vi "Format InstancePrivateIpAddressSetItemType_LVXML.vi"(8 "error in (no error)":errorcluster, 10 "valueXmlData 3":T2, 11 "AWS_EC2 in":refnum<class "AWS_EC2.lvclass">) -> (0 "error out":errorcluster, 2 "Array":T3[](array[typedef]), 3 "AWS_EC2 out":refnum<class "AWS_EC2.lvclass">)   [LabVIEW 2014, in "AWS_EC2.lvlib" / "AWS_EC2.lvclass"]
uses:
  AWS_EC2.lvclass
  EC2 Datatypes/InstancePrivateIpAddressesSetItemType.ctl
  EC2 Datatypes/InstanceNetworkInterfaceAssociationType.ctl
  lv-xml-parser/r0/trunk/VI Source/EventType.ctl
  lv-xml-parser/r0/trunk/VI Source/LV XML Parser.lvlib
  AWS_EC2.lvlib
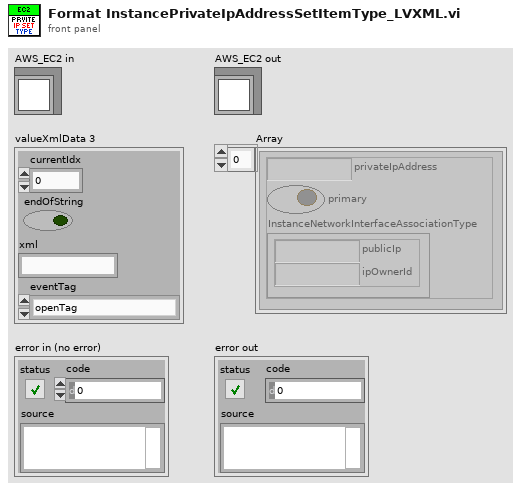
[diagram p1: front panel]
types:
  T1 = typedef "LV XML Parser.lvlib/EventType.ctl" = enum16{"openTag", "endOpenTag", "closeTag", "comment", "endComment", "endOfFile", "attribute", "startXml"}
  T2 = cluster{"currentIdx":i32, "endOfString":bool, "xml":string, "eventTag":T1}
  T3 = typedef "AWS_EC2.lvlib/InstancePrivateIpAddressesSetItemType.ctl" = cluster{"privateIpAddress":string, "primary":bool, "InstanceNetworkInterfaceAssociationType":T4}
  T4 = typedef "AWS_EC2.lvlib/InstanceNetworkInterfaceAssociationType.ctl" = cluster{"publicIp":string, "ipOwnerId":string}
  T5 = cluster{"namespaceUri":string, "localName":string}
  T6 = cluster{"Attributes":cluster{"localName":string, "namespaceUri":string, "value":string}[], "localName":string, "namespaceUri":string, "valueXmlData":cluster{"currentIdx":i32, "endOfString":bool, "xml":string, "eventTag":T1}}[]
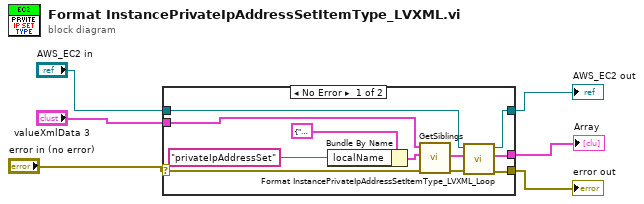
[diagram p0: block diagram]
diagram:
  n1 = case shown="No Error" "error in (no error)" {
    selector: "error in (no error)" -> [w13 w18]
    tunnel: [w9 w19] -> w4
    tunnel: "AWS_EC2 in" -> [w10 w19]
    tunnel: [w7 w18] -> w2
    tunnel: "valueXmlData 3" -> [w17 _]
    tunnel: [w8 _] -> w6
    frame No Error {
      n2 = Bundle By Name(cluster=T5 {"namespaceUri"="", "localName"=""} ("limitToTag"), "localName"="privateIpAddressSet" ("Tag name")) -> (w14:T5)
      n3 = call "GetSiblings.vi"("error in (no error)"=w13, "limitToTag"=w14, "xmlData"=w17) -> ("error out"=w12:errorcluster, "Siblings"=w11:T6)  [unwired: 7 in]
      n4 = call "Format InstancePrivateIpAddressSetItemType_LVXML_Loop.vi"("error in (no error)"=w12, "Siblings in 4"=w11, "AWS_EC2 in"=w10) -> ("error out"=w7:errorcluster, "Array"=w8:T3[], "AWS_EC2 out"=w9:refnum<class "AWS_EC2.lvclass">)  [unwired: 6 in]
    }
    frame Error {
    }
  }
  "Array" <- w6
  "AWS_EC2 out" <- w4
  "error out" <- w2
